vi "Stuckbead Scan and Auto Save_YCC.vi"(8 "File name add to the end":string="h0", 9 "Scan Range  (um)":dbl=2.0 format="%.3f", 10 "Save Data?":bool, 11 "Axis (XYZ)":enum16{"x", "y", "z"}(ring)) -> ()   [LabVIEW 2014]
uses:
  Main-Stage-Based/(Global) Current handle and LaserPower_YCC.vi
  <vilib>/Analysis/polynomials.llb/Scalar Polynomial Evaluation (DBL).vi
  <vilib>/Analysis/NI_AALPro.lvlib
panel:
  in  "Filter type":T1(ring)=enum."Moving-window avg"
  out "delta xBead (nm)":dbl[](array[numeric])
  out "Bead Position (nm)":dbl[](array[numeric])
  in  "Stuckbead path (dialog if empty)":path=path "D:/Calibration-Stuckbead-Scan/20181030/2/034619-x-Stuckbead Scan-20.00-step 5.00 nm-QPD height 0.814-h0.txt"
  in  "Who's Data":T2(ring)
  out "step size (nm)":dbl
  out "QPD height for tether (V)":dbl
  in  "Enum":enum16{"parity method", "max-min method"}(ring)=enum."max-min method"
  in  "waiting time per point (ms)\nrange from 5ms to 0.167 ms":dbl=5.0
  out "mean QPD":dbl
  out "Positon Start scan point (um)":dbl
  out "Filtered QPD data":dbl[](array[numeric])
  out "Filtered Stage Array":dbl[](array[numeric])
  out "Running time":dbl
  in  "Move to new Center?":bool=TRUE
  in  "no record \nscan rate  (um/s)":dbl=4.0
  out "need time":dbl
  out "True rate?":bool
  out "Sample points want to record":dbl
  out "Center (um)":dbl
  out "Move to":dbl
  in  "Tab Control":T3(tab)
  out "Filtered stage-QPD Graph (XY)":T4(graph)
  out "Raw+Filter stage-QPD Graph":cluster{"Raw Stage Array":dbl[], "data":dbl[]}[](graph)
  out "stage-QPD Graph":cluster{"Raw Stage Array":dbl[], "data":dbl[]}[](graph)
  in  "Avg points":i32=620
  out "Stage Array from one end to the other end":dbl[](array[numeric])
  out "total time to travel (s)":dbl
  out "Axis to Read":i32
  in  "T=+ first\nF=- first":bool
  out "Real initial position (um)":dbl format="%0.5f"
  in  "Sampling rate (Hz)":dbl=32000.0 format="%0.2f"
  in  "scan rate  (um/s)":dbl=1.0 format="%.3f"
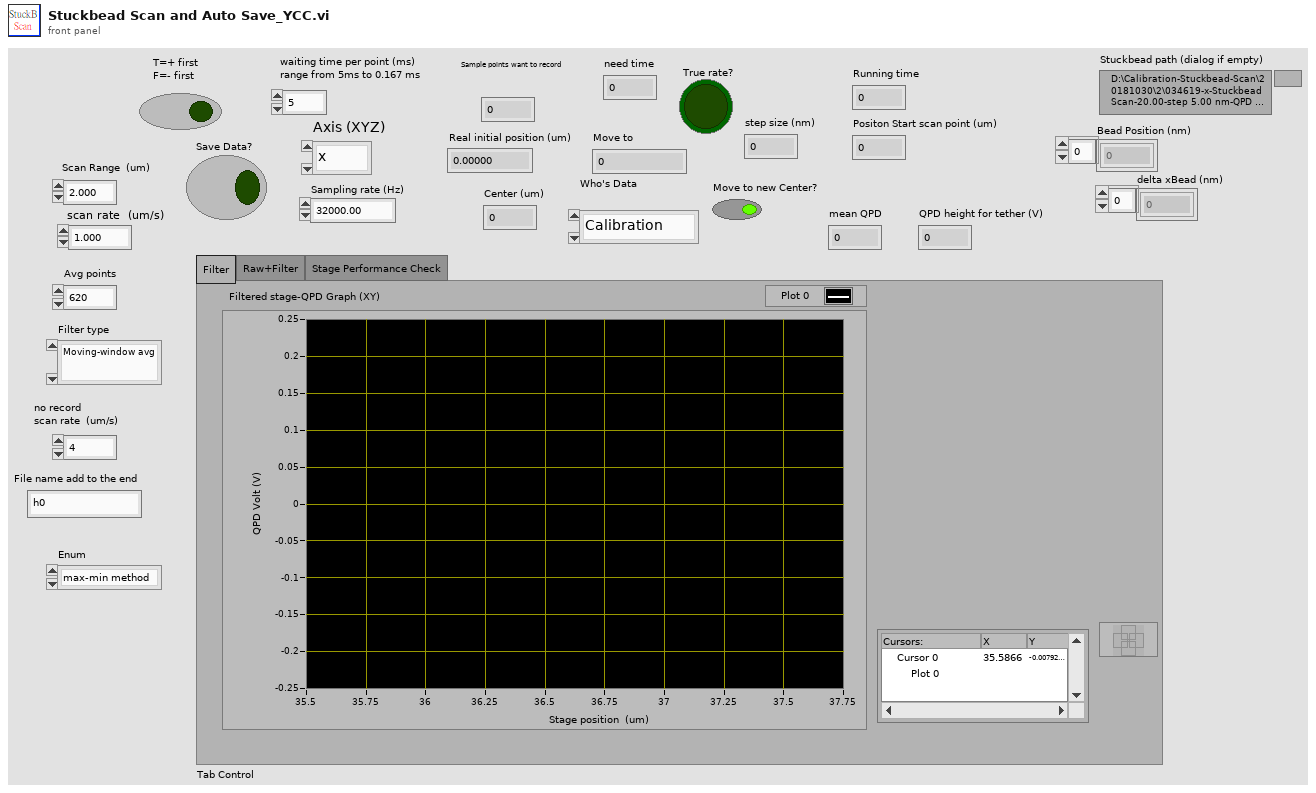
[diagram p1: front panel]
types:
  T1 = enum16{"Fixed-window avg", "Moving-window avg", "F+S-window avg", "S-G filter", "Fixed-window Median", "Moving-window Median "}
  T2 = enum16{"Calibration", "YCC", "PYW", "LCH", "YYH"}
  T3 = enum32{"Filter", "Raw+Filter", "Stage Performance Check"}
  T4 = cluster{"Filtered Stage Array":dbl[], "Another Axis Filt. QPD (X or Y)":dbl[]}[]
  T5 = cluster{"Raw Stage Array":dbl[], "Filtered QPD data out":dbl[]}
  T6 = cluster{"Filtered Stage Array":dbl[], "Filtered QPD data out":dbl[]}
  T7 = cluster{"Filtered Stage Array":dbl[], "Another Axis Filt. QPD (X or Y)":dbl[]}
  T8 = cluster{"Raw Stage Array":dbl[], "Filtered QPD data out":dbl[]}[]
  T9 = cluster{"stuckbead-QPD (V)":dbl[], "Bead radius (nm)":dbl[]}[]
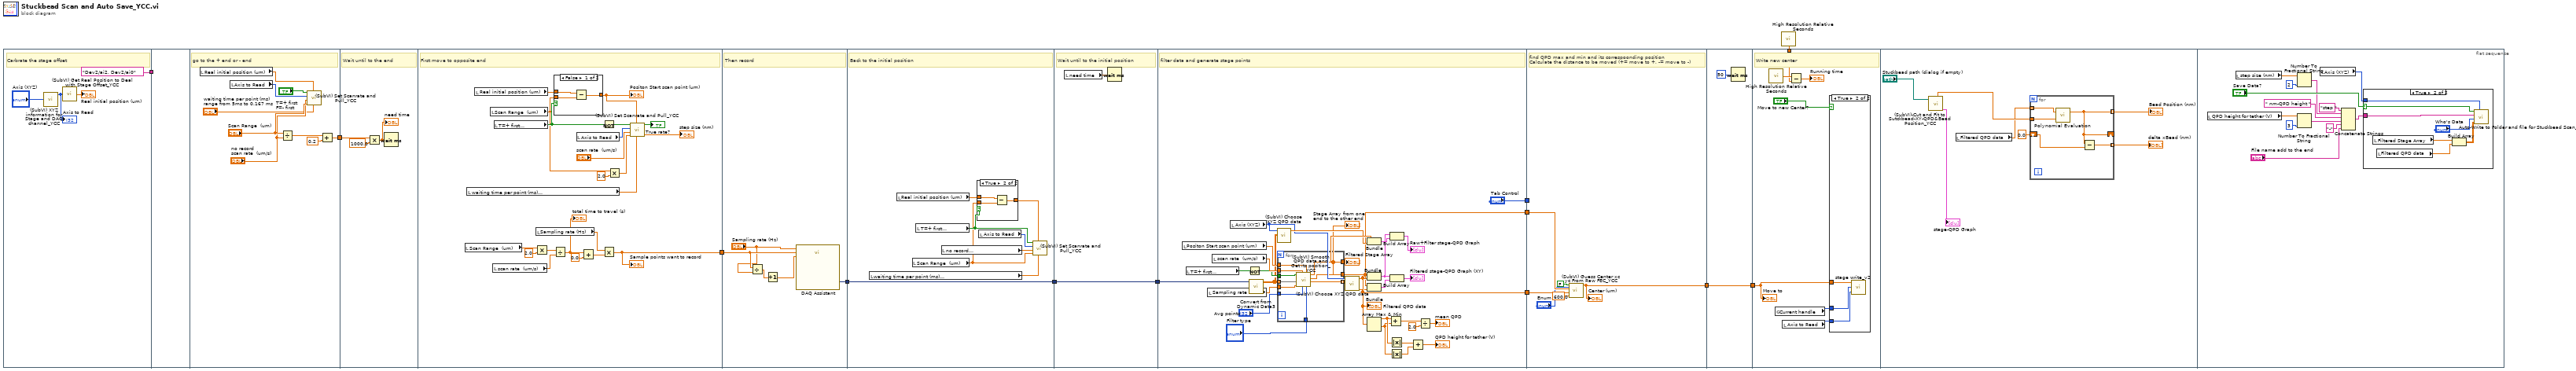
[diagram p0: block diagram]
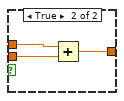
[diagram p2: hidden frame]
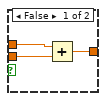
[diagram p3: hidden frame]
diagram:
  n1 = flat-sequence {
    tunnel: [tag "Dev2/ai2, Dev2/ai0" ("physical channels")] -> w12
    tunnel: w12 -> [_]
    tunnel: [w21] -> w8
    tunnel: w8 -> [w28]
    tunnel: [w37] -> w5
    tunnel: [w60] -> w7
    tunnel: w5 -> [w59]
    tunnel: w7 -> [w68]
    tunnel: [w68] -> w6
    tunnel: w6 -> [w75]
    tunnel: [w75] -> w1
    tunnel: [w89] -> w11
    tunnel: [w86] -> w10
    tunnel: ["Tab Control"] -> w9
    tunnel: w1 -> [w79]
    tunnel: w11 -> [w119]
    tunnel: w10 -> [w122]
    tunnel: w9 -> [_]
    tunnel: [w118] -> w2
    tunnel: [w123] -> w3
    tunnel: w2 -> [w123]
    tunnel: w4 -> [w127]
    tunnel: w3 -> [w125]
    frame #0 {
      # "Carbrate the stage offset"
      n2 = call "(SubVI) XYZ information for Stage and DAQ channel_YCC.vi"("Axis  (Enum)"="Axis (XYZ)") -> ("Axis"=w13:i32)  [unwired: 3 in, 1 out]
      "Axis to Read" <- w13
      n3 = call "(SubVI) Get Real Position to Deal with Stage Offset_YCC.vi"("Axis"=w13) -> ("Real Current Commanded position (um)"=→"Real initial position (um)":dbl)  [unwired: 3 in, 1 out]
    }
    frame #1 {
    }
    frame #2 {
      # "go to the + end or - end"
      n4 = local read "Real initial position (um)"() -> (w19:dbl)
      n5 = local read "Axis to Read"() -> (w25:i32)
      n6 = Divide(x="Scan Range  (um)", y="no record \nscan rate  (um/s)") -> (x/y=w23:dbl)
      n7 = call "(SubVI) Set Scanrate and Pull_YCC.vi"("toward+ ?\nT=+, F=-"="T=+ first\nF=- first", "Start From  (um)"=w19, "axis"=w25, "scan rate  (um/s)"="no record \nscan rate  (um/s)", "waiting time per point (ms)\nrange from 5ms to 0.167 ms"="waiting time per point (ms)\nrange from 5ms to 0.167 ms", "range  (um)"="Scan Range  (um)") -> ()  [unwired: 3 out]
      n8 = Add(x=w23, y=0.2) -> (x+y=w21:dbl)
    }
    frame #3 {
      # "Wait until to the end"
      n9 = Multiply(x=w28, y=1000.0) -> (x*y=w26:dbl)
      "need time" <- w26
      n10 = Wait (ms)(milliseconds to wait=w26) -> ()  [unwired: 1 out]
    }
    frame #4 {
      # "First move to opposite end"
      n11 = local read "Scan Range  (um)"() -> (w39:dbl)
      n12 = local read "waiting time per point (ms)\nrange from 5ms to 0.167 ms"() -> (w30:dbl)
      n13 = local read "Real initial position (um)"() -> (w34:dbl)
      n14 = local read "Scan Range  (um)"() -> (w33:dbl)
      n15 = local read "scan rate  (um/s)"() -> (w38:dbl)
      n16 = local read "T=+ first\nF=- first"() -> (w35:bool)
      n17 = Multiply(x=w39, y=2.0) -> (x*y=w41:dbl)
      n18 = local read "Sampling rate (Hz)"() -> (w31:dbl)
      n19 = Divide(x=w41, y=w38) -> (x/y=w42:dbl)
      "total time to travel (s)" <- w42
      n20 = case shown="False" w35 {
        tunnel: w34 -> [w52 w55]
        tunnel: w33 -> [w51 w54]
        tunnel: [w50 w53] -> w32
        frame False {
          n21 = Subtract(x=w52, y=w51) -> (x-y=w50:dbl)
        }
        frame True {
          n22 = Add(x=w55, y=w54) -> (x+y=w53:dbl)
        }
      }
      "Positon Start scan point (um)" <- w32
      n23 = local read "Axis to Read"() -> (w36:i32)
      n24 = Add(x=w42, y=0.0) -> (x+y=w43:dbl)
      n25 = Not(x=w35) -> (.not. x?=w45:bool)
      n26 = Multiply(x=w31, y=w43) -> (x*y=w37:dbl)
      "Sample points want to record" <- w37
      n27 = Multiply(x=w33, y=2.0) -> (x*y=w46:dbl)
      n28 = call "(SubVI) Set Scanrate and Pull_YCC.vi"("toward+ ?\nT=+, F=-"=w45, "Start From  (um)"=w32, "axis"=w36, "scan rate  (um/s)"="scan rate  (um/s)", "waiting time per point (ms)\nrange from 5ms to 0.167 ms"=w30, "range  (um)"=w46) -> ("True rate?"=→"True rate?":bool, "step size (nm)"=→"step size (nm)":dbl)  [unwired: 1 out]
    }
    frame #5 {
      # "Then record"
      n29 = Divide(x=w59, y="Sampling rate (Hz)") -> (x/y=w57:dbl)
      n30 = Increment(x=w57) -> (x+1=w56:dbl)
      n31 = call "DAQ Assistant"("rate"="Sampling rate (Hz)", "number of samples"=w59, "timeout (s)"=w56) -> ("data"=w60:dynamicdata)  [unwired: 14 in, 2 out]
    }
    frame #6 {
      # "Back to the initial position"
      n32 = local read "waiting time per point (ms)\nrange from 5ms to 0.167 ms"() -> (w61:dbl)
      n33 = local read "Real initial position (um)"() -> (w64:dbl)
      n34 = local read "Scan Range  (um)"() -> (w63:dbl)
      n35 = local read "T=+ first\nF=- first"() -> (w65:bool)
      n36 = local read "no record \nscan rate  (um/s)"() -> (w67:dbl)
      n37 = case shown="True" w65 {
        tunnel: [w71 w74] -> w62
        tunnel: w64 -> [w70 w73]
        tunnel: w63 -> [w69 w72]
        frame False {
          n38 = Add(x=w70, y=w69) -> (x+y=w71:dbl)
        }
        frame True {
          n39 = Subtract(x=w73, y=w72) -> (x-y=w74:dbl)
        }
      }
      n40 = local read "Axis to Read"() -> (w66:i32)
      n41 = call "(SubVI) Set Scanrate and Pull_YCC.vi"("toward+ ?\nT=+, F=-"=w65, "Start From  (um)"=w62, "axis"=w66, "scan rate  (um/s)"=w67, "waiting time per point (ms)\nrange from 5ms to 0.167 ms"=w61, "range  (um)"=w63) -> ()  [unwired: 3 out]
    }
    frame #7 {
      # "Wait until to the initial position"
      n42 = local read "need time"() -> (w76:dbl)
      n43 = Wait (ms)(milliseconds to wait=w76) -> ()  [unwired: 1 out]
    }
    frame #8 {
      # "filter data and generate stage points"
      n44 = local read "Positon Start scan point (um)"() -> (w98:dbl)
      n45 = local read "T=+ first\nF=- first"() -> (w100:bool)
      n46 = local read "Sampling rate (Hz)"() -> (w105:dbl)
      n47 = local read "scan rate  (um/s)"() -> (w104:dbl)
      n48 = local read "Axis (XYZ)"() -> (w84:enum16{"x", "y", "z"})
      n49 = Not(x=w100) -> (.not. x?=w99:bool)
      n50 = call "Convert from Dynamic Data3"("Dynamic Data Type"=w79) -> ("Array"=w78:dbl[][])  [unwired: 3 in]
      n51 = call "(SubVI) Choose XYZ QPD data.vi"("Filtered QPD data in"=w78, "Axis"=w84) -> ("Filtered QPD data out"=w88:dbl[])  [unwired: 8 in, 1 out]
      n52 = for {
        tunnel: w105 -> [w116]
        tunnel: w104 -> [w115]
        tunnel: "Avg points" -> [w114]
        tunnel: [w113] -> w86
        tunnel: [w112] -> w102
        tunnel: w99 -> [w111]
        tunnel: w98 -> [w110]
        tunnel: [w109] -> w85 mode=indexing
        tunnel: w78 -> [w108] mode=indexing
        tunnel: "Filter type" -> [w107]
        n53 = call "(SubVI) Smooth QPD data and Get its position_YCC.vi"("Filter type"=w107, "Initial position (um)"=w110, "Avg points"=w114, "scan rate  (um/s)"=w115, "Sampling rate (Hz)"=w116, "QPD data"=w108, "Direction\nT=+ \nF=-"=w111) -> ("Filtered QPD data"=w109:dbl[], "Filtered Stage Array"=w113:dbl[], "Raw Stage Array"=w112:dbl[])  [unwired: 2 in]
      }
      "Stage Array from one end to the other end" <- w86
      "Filtered Stage Array" <- w86
      n54 = call "(SubVI) Choose XYZ QPD data.vi"("Filtered QPD data in"=w85, "Axis"=w84) -> ("Another Axis Filt. QPD (X or Y)"=w83:dbl[], "Filtered QPD data out"=w89:dbl[])  [unwired: 8 in]
      "Filtered QPD data" <- w89
      n55 = Bundle("Raw Stage Array"=w102, "Filtered QPD data out"=w88) -> (w87:T5)  [unwired: 1 in]
      n56 = Bundle("Filtered Stage Array"=w86, "Filtered QPD data out"=w89) -> (w82:T6)  [unwired: 1 in]
      n57 = Bundle("Filtered Stage Array"=w86, "Another Axis Filt. QPD (X or Y)"=w83) -> (w81:T7)  [unwired: 1 in]
      n58 = Array Max & Min(array=w89) -> (max value=w94:dbl, min value=w93:dbl)  [unwired: 2 out]
      n59 = Add(x=w94, y=w93) -> (x+y=w97:dbl)
      n60 = Build Array(w82, w87) -> (→"Raw+Filter stage-QPD Graph":T8)
      n61 = Build Array(w82, w81) -> (→"Filtered stage-QPD Graph (XY)":T4)
      n62 = Absolute Value(x=w94) -> (abs(x)=w92:dbl)
      n63 = Absolute Value(x=w93) -> (abs(x)=w91:dbl)
      n64 = Add(x=w92, y=w91) -> (x+y=→"QPD height for tether (V)":dbl)
      n65 = Divide(x=w97, y=2.0) -> (x/y=→"mean QPD":dbl)
    }
    frame #9 {
      # "find QPD max and min and its correspoonding position\nCalculate the distance to be moved (+= move to +, -= move to -)"
      n66 = call "(SubVI) Guess Center xc yc From Raw FEC_YCC.vi"("Enum"="Enum", "avg range for QPD center (nm)"=600.0, "QPD array (V)"=w119, "Stage array(um)"=w122, "Read data?"=FALSE) -> ("Guess-stage-center(um)"=w118:dbl)  [unwired: 1 in, 3 out]
      "Center (um)" <- w118
    }
    frame #10 {
      n67 = Wait (ms)(milliseconds to wait=u32 50) -> ()  [unwired: 1 out]
    }
    frame #11 {
      # "Write new center"
      n68 = call <vilib>:"High Resolution Relative Seconds.vi"() -> ("relative seconds"=w128:dbl)
      n69 = global read "(Global) Current handle and LaserPower_YCC.vi" "Current handle"() -> (w130:i32)
      n70 = local read "Axis to Read"() -> (w129:i32)
      n71 = Subtract(x=w128, y=w127) -> (x-y=→"Running time":dbl)
      n72 = case shown="True" "Move to new Center?" {
        tunnel: w125 -> [_ w134]
        tunnel: w130 -> [_ w133]
        tunnel: w129 -> [_ w132]
        frame False {
        }
        frame True {
          n73 = call "stage write_v2.vi"("axis"=w132, "Incoming Handle"=w133, "position"=w134) -> ()  [unwired: 2 in, 1 out]
        }
      }
      "Move to" <- w125
    }
    frame #12 {
      n74 = call "(SubVI)-Cut and Fit to Sutckbead-XY-QPD&BeadPosition_YCC.vi"("Stuckbead path (dialog if empty)"="Stuckbead path (dialog if empty)") -> ("All fig"=→"stage-QPD Graph":T9, "Polynomial Coefficients\nx:QPD, y:BeadPos"=w139:dbl[])  [unwired: 2 in, 3 out]
      n75 = local read "Filtered QPD data"() -> (w138:dbl[])
      n76 = for {
        tunnel: w139 -> [w146]
        tunnel: w138 -> [w145] mode=indexing
        tunnel: [w144] -> w137 mode=indexing
        shift-right: [w144] -> _
        shift-left: 0.0 ("P(a)") -> [w143]
        tunnel: [w142] -> w136 mode=indexing
        n77 = call-poly <vilib>:"Polynomial Evaluation.vi"("P(x)"=w146, "a"=w145) -> ("P(a)"=w144:dbl)  [unwired: 1 out]
        n78 = Subtract(x=w144, y=w143) -> (x-y=w142:dbl)
      }
      "Bead Position (nm)" <- w137
      "delta xBead (nm)" <- w136
    }
    frame #13 {
      n79 = local read "QPD height for tether (V)"() -> (w152:dbl)
      n80 = local read "step size (nm)"() -> (w158:dbl)
      n81 = Number To Fractional String(number=w158, precision (6)=i16 2) -> (F-format string=w154:string)  [unwired: 2 in]
      n82 = Number To Fractional String(number=w152, precision (6)=i16 3) -> (F-format string=w150:string)  [unwired: 2 in]
      n83 = local read "Axis (XYZ)"() -> (w149:enum16{"x", "y", "z"})
      n84 = Concatenate Strings("step " ("string"), w154, " nm-QPD height " ("string"), w150, "-" ("string"), "File name add to the end") -> (w153:string)
      n85 = case shown="True" "Save Data?" {
        selector: "Save Data?" -> [_ w164]
        tunnel: w153 -> [_ w160]
        tunnel: w149 -> [_ w161]
        frame False {
        }
        frame True {
          n86 = local read "Filtered Stage Array"() -> (w166:dbl[])
          n87 = local read "Filtered QPD data"() -> (w165:dbl[])
          n88 = Build Array(w166, w165) -> (w163:dbl[][])
          n89 = call "Auto-Write to Folder and file for Stuckbead Scan_YCC.vi"("Axis (Enum)"=w161, "data to be saved"=w163, "Who's Data"="Who's Data", "File name add to the end"=w160, "Save?"=w164) -> ()  [unwired: 3 in, 2 out]
        }
      }
    }
  }
  n90 = call <vilib>:"High Resolution Relative Seconds.vi"() -> ("relative seconds"=w4:dbl)
